vi "quiz3.4.vi"() -> ()   [LabVIEW 2017]
panel:
  out "Tab Control 2":enum32{"Login", "Menu", "Add", "delete"}(tab)
  in  "Ingresar 2":bool
  in  "Contraseña 2":string
  in  "Usuario 2":string
  in  "Delete Button 2":bool
  in  "Add Button 2":bool
  in  "Home Button 2":bool
  out "Cusuario 2":string
  in  "Previous Button 3":bool
  in  "AddContraseña 2":string
  in  "AddUsuario 2":string
  in  "Agregar 2":bool
  out "Agregado 2":bool
  in  "Cancel Button 2":bool
  in  "DeleteUsuario 3":string
  in  "Previous Button 4":bool
  out "text 2":string
  out "Tab Control":enum32{"Login", "Menu", "Add", "delete"}(tab)
  in  "Ingresar":bool
  in  "Contraseña":string
  in  "Usuario":string
  in  "Delete Button":bool
  in  "Add Button":bool
  in  "Home Button":bool
  out "Cusuario":string
  in  "Previous Button":bool
  in  "AddContraseña":string
  in  "AddUsuario":string
  in  "Agregar":bool
  out "Agregado":bool
  in  "Cancel Button":bool
  in  "DeleteUsuario":string
  in  "Previous Button 2":bool
  out "text":string
  # "USTED INGRESO CON EL USUARIO"
  # "USTED INGRESO CON EL USUARIO"
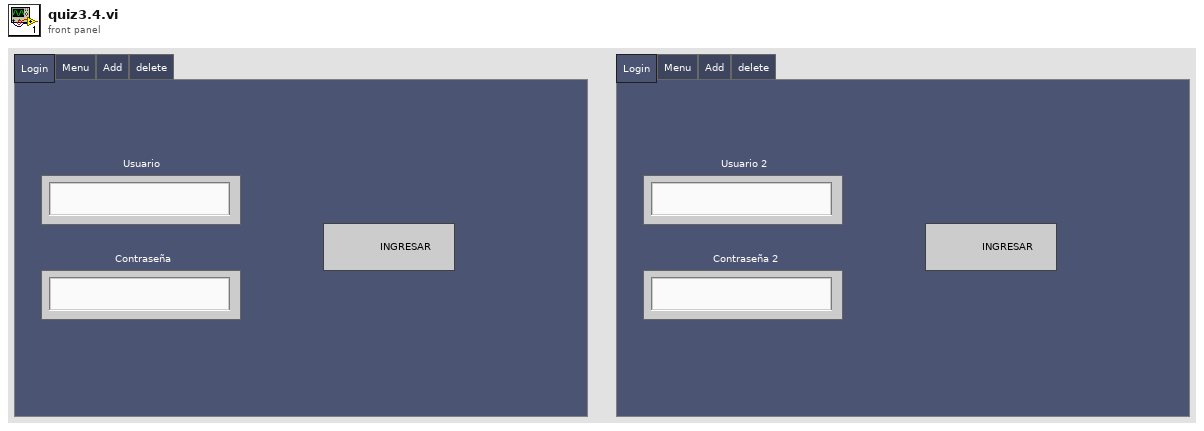
[diagram p1: front panel]
types:
  T1 = enum16{"open", "replace", "create", "open or create", "replace or create", "replace or create with confirmation"}
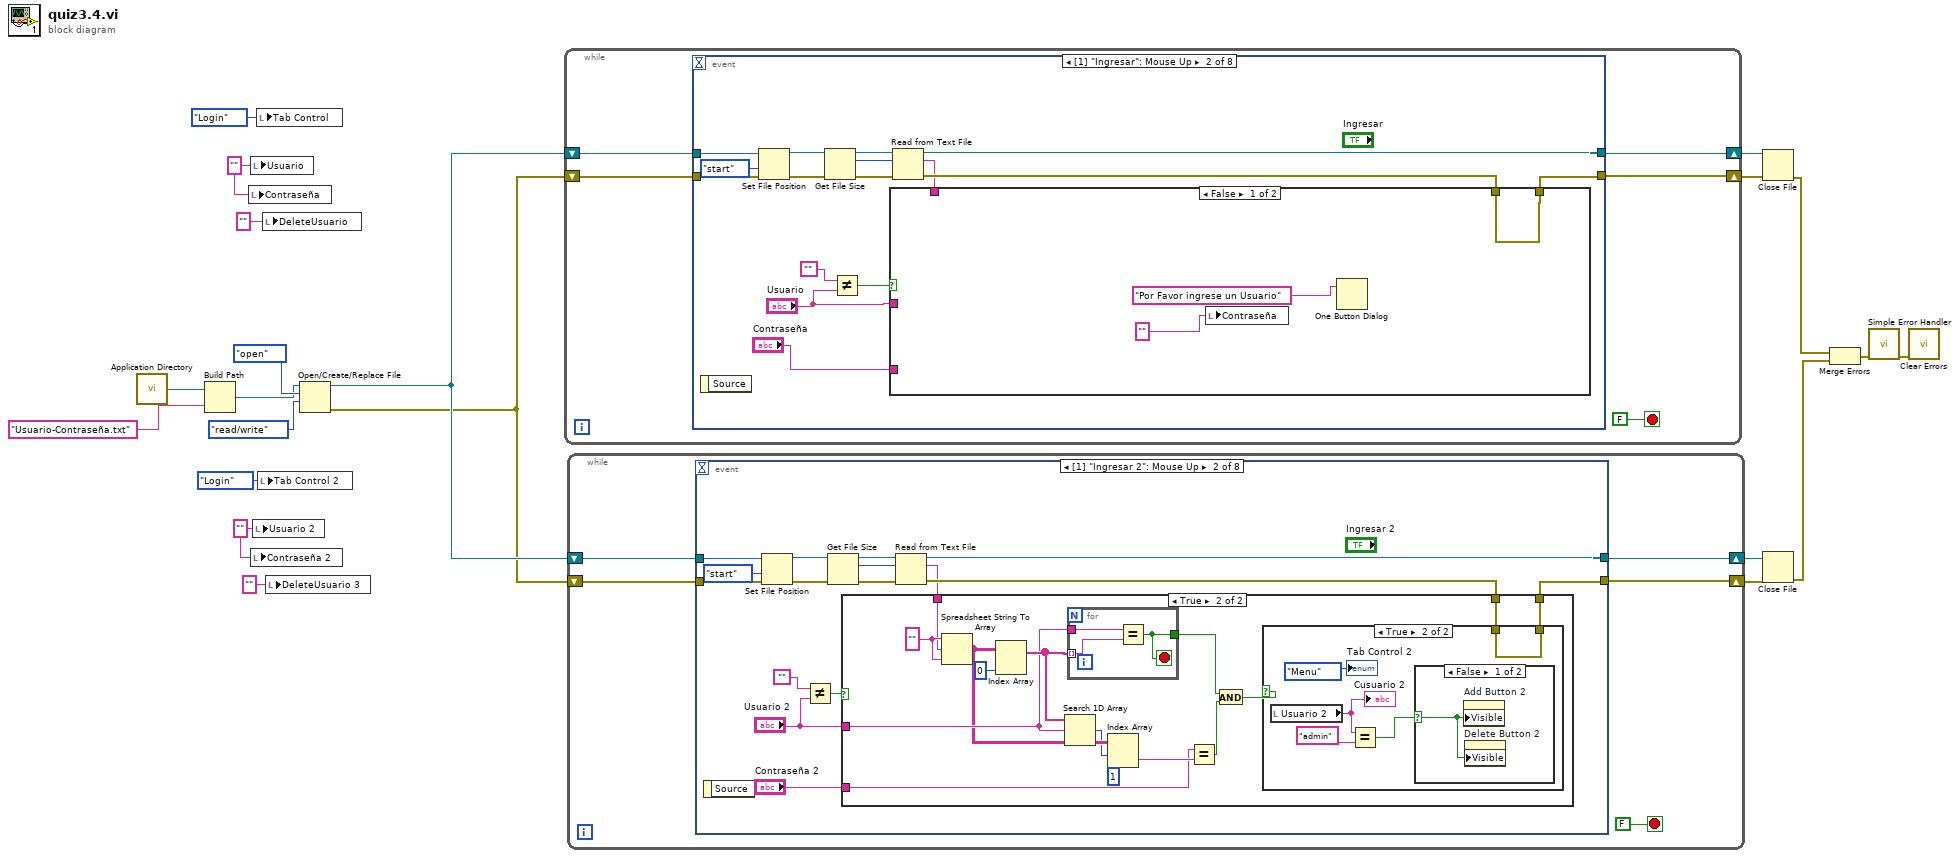
[diagram p0: block diagram]
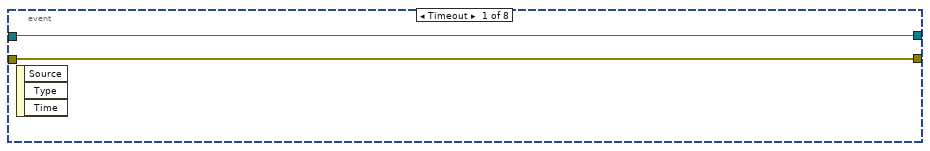
[diagram p2: hidden frame]
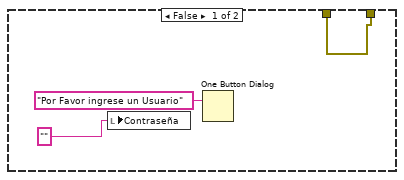
[diagram p3: hidden frame]
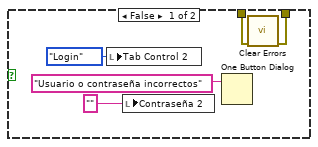
[diagram p4: hidden frame]
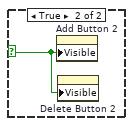
[diagram p5: hidden frame]
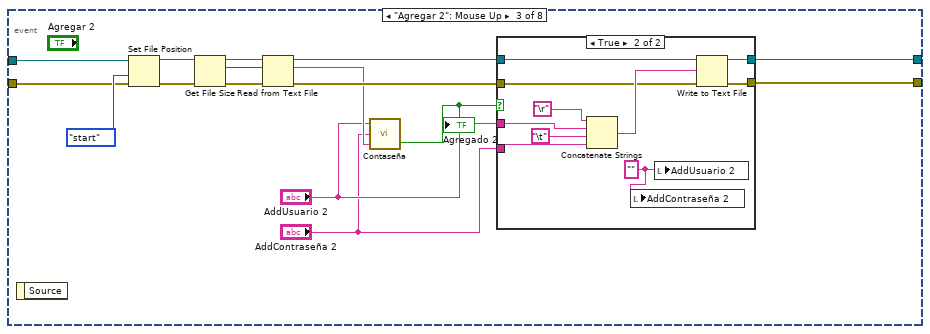
[diagram p6: hidden frame]
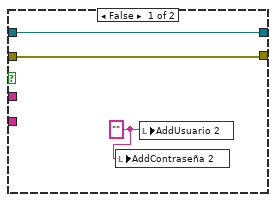
[diagram p7: hidden frame]
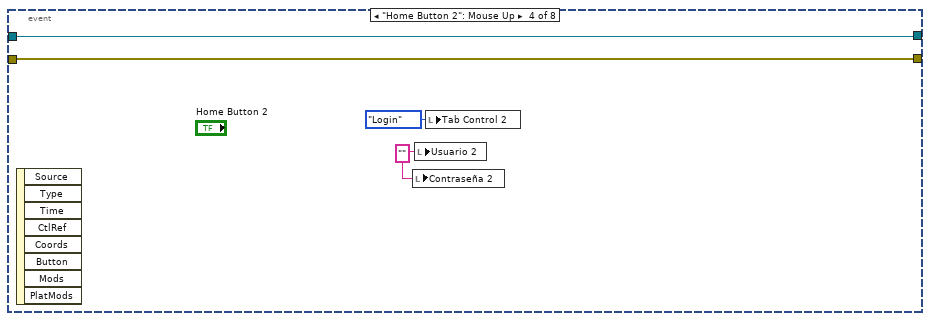
[diagram p8: hidden frame]
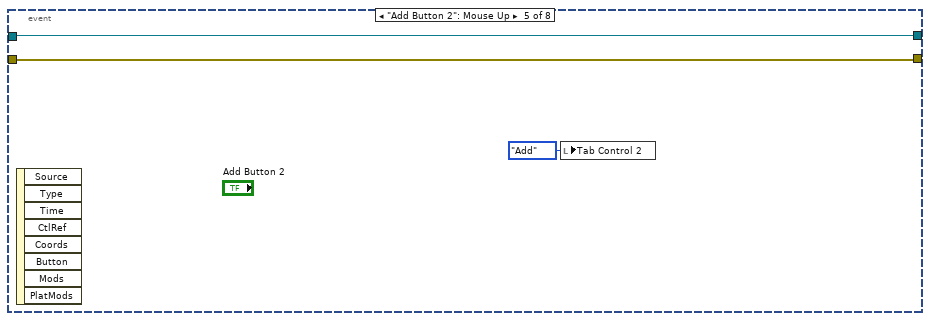
[diagram p9: hidden frame]
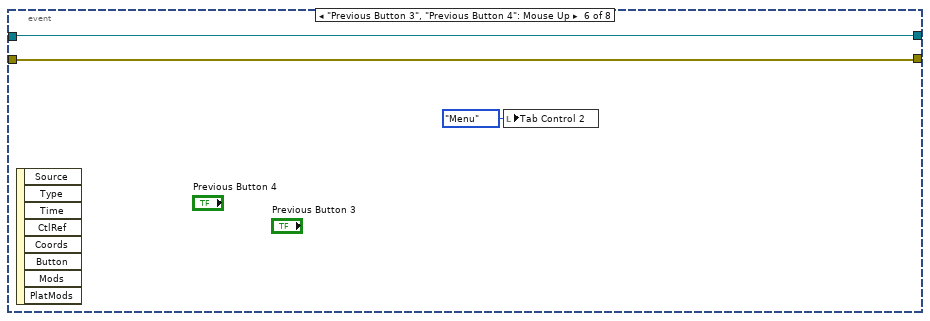
[diagram p10: hidden frame]
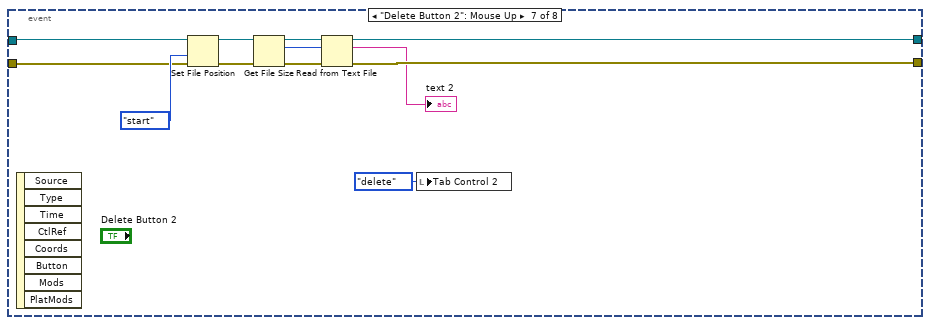
[diagram p11: hidden frame]
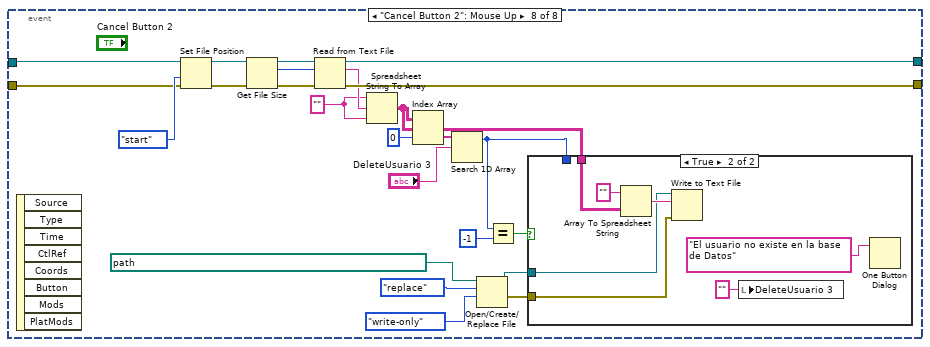
[diagram p12: hidden frame]
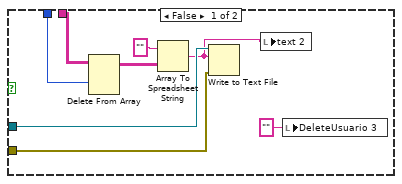
[diagram p13: hidden frame]
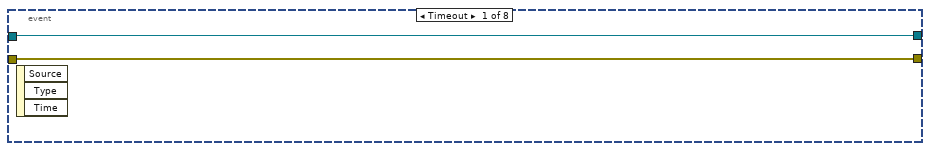
[diagram p14: hidden frame]
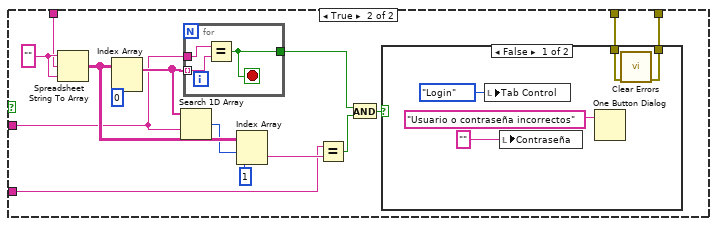
[diagram p15: hidden frame]
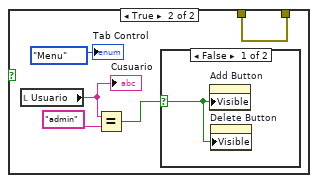
[diagram p16: hidden frame]
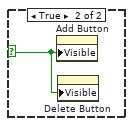
[diagram p17: hidden frame]
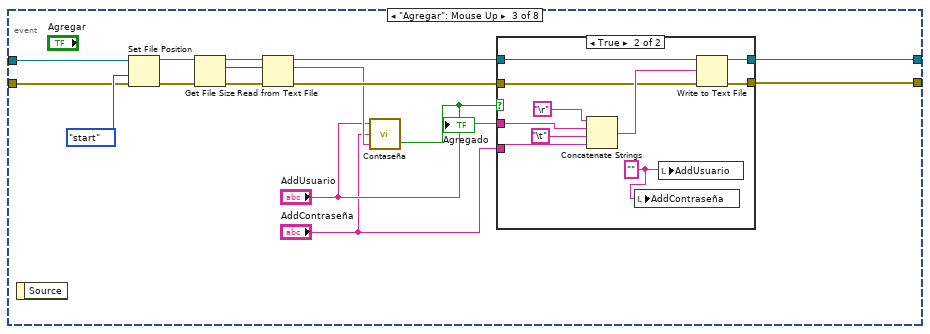
[diagram p18: hidden frame]
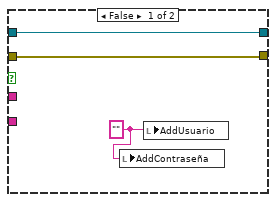
[diagram p19: hidden frame]
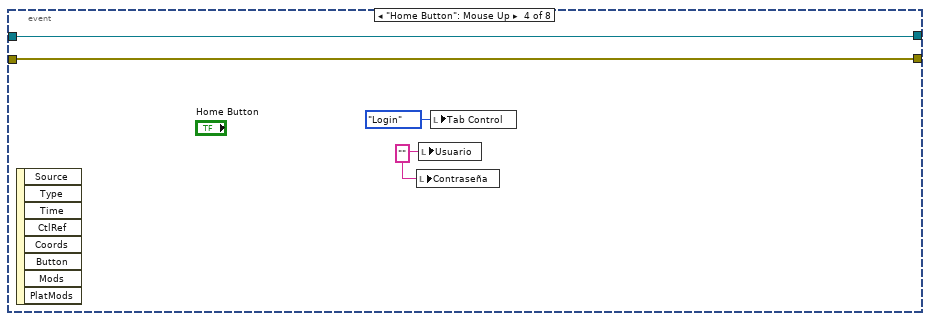
[diagram p20: hidden frame]
diagram:
  w1 = "" ("Usuario")
  w14 = "" ("Usuario")
  n1 = call <vilib>:"Application Directory.vi"() -> ("Application Directory"=w21:path)
  n2 = Build Path(base path=w21, name or relative path="Usuario-Contraseña.txt") -> (appended path=w15:path)
  n3 = local write "Contraseña"(w14) -> ()
  n4 = local write "Usuario"(w14) -> ()
  n5 = local write "Contraseña 2"(w1) -> ()
  n6 = local write "Usuario 2"(w1) -> ()
  n7 = local write "Tab Control"(enum32{"Login", "Menu", "Add", "delete"}."Login" ("Tab Control")) -> ()
  n8 = local write "Tab Control 2"(enum32{"Login", "Menu", "Add", "delete"}."Login" ("Tab Control")) -> ()
  n9 = local write "DeleteUsuario"("" ("DeleteUsuario 2")) -> ()
  n10 = local write "DeleteUsuario 3"("" ("DeleteUsuario 2")) -> ()
  n11 = Open/Create/Replace File(file path (use dialog)=w15, operation (0:open)=T1."open", access (0:read/write)=enum16{"read/write", "read-only", "write-only"}."read/write") -> (refnum out=w5:refnum<file>, error out=w4:errorcluster)  [unwired: 3 in, 1 out]
  n12 = while {
    shift-right: [w23] -> w11
    shift-left: w5 -> [w24]
    shift-right: [w22] -> w16
    shift-left: w4 -> [w25]
    stop <- FALSE stop-if-true
    n13 = event shown="[1] \"Ingresar\": Mouse Up" {
      selector: _ -> [_ _ _ _ _ _ _ _]
      dyn-events: _ -> [_ _ _ _ _ _ _ _]
      timeout: _ -> [_ _ _ _ _ _ _ _]
      tunnel: w25 -> [w27 w44 w81 w108 w112 w115 w119 w146]
      tunnel: [w28 w39 w93 w109 w113 w116 w120 w142] -> w23
      tunnel: [w27 w36 w92 w108 w112 w115 w118 w141] -> w22
      tunnel: w24 -> [w28 w38 w82 w109 w113 w116 w121 w145]
      event Timeout {
        n14 = event-data() -> ()  [unwired: 1 in, 3 out]
      }
      event "Ingresar": Mouse Up {
        n15 = event-data() -> ()  [unwired: 1 in, 1 out]
        n16 = Set File Position(refnum=w38, from (0:start)=enum16{"start", "end", "current"}."start", error in=w44) -> (refnum out=w42:refnum<file>, error out=w43:errorcluster)  [unwired: 1 in]
        n17 = Get File Size(file=w42, error in=w43) -> (refnum out=w34:refnum<file>, size (in bytes)=w41:i64, 0:w40:errorcluster)
        n18 = Not Equal?(x="", y="Usuario") -> (x != y?=w31:bool)
        n19 = Read from Text File(file (use dialog)=w34, count=w41, error in=w40) -> (refnum out=w39:refnum<file>, text=w33:string, error out=w37:errorcluster)  [unwired: 1 in, 1 out]
        n20 = case shown="False" w31 {
          tunnel: w37 -> [w47 w62]
          tunnel: [w47 w61] -> w36
          tunnel: w33 -> [_ w58]
          tunnel: "Usuario" -> [_ w49]
          tunnel: "Contraseña" -> [_ w48]
          frame False {
            n21 = local write "Contraseña"("" ("Usuario")) -> ()
            n22 = One Button Dialog(message="Por Favor ingrese un Usuario") -> ()  [unwired: 1 in, 1 out]
          }
          frame True {
            w59 = "" ("format string")
            n23 = Spreadsheet String To Array(format string=w59, spreadsheet string=w58, array type (2D Dbl)=w59) -> (array=w55:string[][])  [unwired: 1 in]
            n24 = Index Array(array=w55, index (col)=0 ("index")) -> (element=w56:string[])  [unwired: 1 in]
            n25 = Search 1D Array(1D array=w56, element=w49) -> (index of element=w52:i32)  [unwired: 1 in]
            n26 = for {
              tunnel: [w65] -> w57
              tunnel: w56 -> [w64] mode=indexing
              tunnel: w49 -> [w63]
              stop <- w65 stop-if-true
              n27 = Equal?(x=w63, y=w64) -> (x = y?=w65:bool)
            }
            n28 = Index Array(array=w55, index (row)=w52, index (col)=1 ("index")) -> (element=w50:string)
            n29 = Equal?(x=w48, y=w50) -> (x = y?=w54:bool)
            n30 = And(x=w57, y=w54) -> (x .and. y?=w60:bool)
            n31 = case shown="False" w60 {
              tunnel: [w68 w75] -> w61
              tunnel: w62 -> [w67 w75]
              frame False {
                n32 = local write "Tab Control"(enum32{"Login", "Menu", "Add", "delete"}."Login" ("Tab Control")) -> ()
                n33 = local write "Contraseña"("" ("Usuario")) -> ()
                n34 = One Button Dialog(message="Usuario o contraseña incorrectos") -> ()  [unwired: 1 in, 1 out]
                n35 = call <vilib>:"Clear Errors.vi"("error in (no error)"=w67) -> ("error out"=w68:errorcluster)  [unwired: 5 in, 1 out]
              }
              frame True {
                n36 = local read "Usuario"() -> (w73:string)
                "Cusuario" <- w73
                n37 = Equal?(x=w73, y="admin") -> (x = y?=w74:bool)
                n38 = case shown="False" w74 {
                  selector: w74 -> [w76 w77]
                  frame False {
                    n39 = property on="Add Button" class="Bool (strict)"("Visible"=w76) -> ()  [unwired: 2 in, 2 out]
                    n40 = property on="Delete Button" class="Bool (strict)"("Visible"=w76) -> ()  [unwired: 2 in, 2 out]
                  }
                  frame True {
                    n41 = property on="Add Button" class="Bool (strict)"("Visible"=w77) -> ()  [unwired: 2 in, 2 out]
                    n42 = property on="Delete Button" class="Bool (strict)"("Visible"=w77) -> ()  [unwired: 2 in, 2 out]
                  }
                }
                "Tab Control" <- enum32{"Login", "Menu", "Add", "delete"}."Menu" ("Tab Control")
              }
            }
          }
        }
      }
      event "Agregar": Mouse Up {
        n43 = event-data() -> ()  [unwired: 1 in, 1 out]
        n44 = Set File Position(refnum=w82, from (0:start)=enum16{"start", "end", "current"}."start", error in=w81) -> (refnum out=w89:refnum<file>, error out=w90:errorcluster)  [unwired: 1 in]
        n45 = Get File Size(file=w89, error in=w90) -> (refnum out=w86:refnum<file>, size (in bytes)=w88:i64, 0:w87:errorcluster)
        n46 = Read from Text File(file (use dialog)=w86, count=w88, error in=w87) -> (refnum out=w84:refnum<file>, text=w80:string, error out=w83:errorcluster)  [unwired: 1 in, 1 out]
        n47 = call "Contaseña.vi"("spreadsheet string"=w80, "AddContraseña"="AddContraseña", "addUsuario"="AddUsuario") -> ("result"=w91:bool)  [unwired: 1 out]
        "Agregado" <- w91
        n48 = case shown="True" w91 {
          tunnel: [w96 w106] -> w93
          tunnel: [w95 w105] -> w92
          tunnel: w84 -> [w96 w101]
          tunnel: w83 -> [w95 w100]
          tunnel: "AddUsuario" -> [_ w99]
          tunnel: "AddContraseña" -> [_ w98]
          frame False {
            w94 = "" ("Usuario")
            n49 = local write "AddContraseña"(w94) -> ()
            n50 = local write "AddUsuario"(w94) -> ()
          }
          frame True {
            w97 = "" ("Usuario")
            n51 = Concatenate Strings("\r", w99, "\t", w98) -> (w104:string)
            n52 = local write "AddContraseña"(w97) -> ()
            n53 = local write "AddUsuario"(w97) -> ()
            n54 = Write to Text File(file (use dialog)=w101, text=w104, error in=w100) -> (refnum out=w106:refnum<file>, error out=w105:errorcluster)  [unwired: 1 in, 1 out]
          }
        }
      }
      event "Home Button": Mouse Up {
        w110 = "" ("Usuario")
        n55 = event-data() -> ()  [unwired: 1 in, 8 out]
        n56 = local write "Contraseña"(w110) -> ()
        n57 = local write "Usuario"(w110) -> ()
        n58 = local write "Tab Control"(enum32{"Login", "Menu", "Add", "delete"}."Login" ("Tab Control")) -> ()
      }
      event "Add Button": Mouse Up {
        n59 = event-data() -> ()  [unwired: 1 in, 8 out]
        n60 = local write "Tab Control"(enum32{"Login", "Menu", "Add", "delete"}."Add" ("Tab Control")) -> ()
      }
      event "Previous Button", "Previous Button 2": Mouse Up {
        n61 = event-data() -> ()  [unwired: 1 in, 8 out]
        n62 = local write "Tab Control"(enum32{"Login", "Menu", "Add", "delete"}."Menu" ("Tab Control")) -> ()
      }
      event "Delete Button": Mouse Up {
        n63 = event-data() -> ()  [unwired: 1 in, 8 out]
        n64 = Set File Position(refnum=w121, from (0:start)=enum16{"start", "end", "current"}."start", error in=w119) -> (refnum out=w126:refnum<file>, error out=w127:errorcluster)  [unwired: 1 in]
        n65 = Get File Size(file=w126, error in=w127) -> (refnum out=w123:refnum<file>, size (in bytes)=w125:i64, 0:w124:errorcluster)
        n66 = Read from Text File(file (use dialog)=w123, count=w125, error in=w124) -> (refnum out=w120:refnum<file>, text=→"text":string, error out=w118:errorcluster)  [unwired: 1 in, 1 out]
        n67 = local write "Tab Control"(enum32{"Login", "Menu", "Add", "delete"}."delete" ("Tab Control")) -> ()
      }
      event "Cancel Button": Mouse Up {
        w138 = "" ("format string")
        n68 = event-data() -> ()  [unwired: 1 in, 8 out]
        n69 = Set File Position(refnum=w145, from (0:start)=enum16{"start", "end", "current"}."start", error in=w146) -> (refnum out=w151:refnum<file>, error out=w152:errorcluster)  [unwired: 1 in]
        n70 = Get File Size(file=w151, error in=w152) -> (refnum out=w148:refnum<file>, size (in bytes)=w150:i64, 0:w149:errorcluster)
        n71 = Read from Text File(file (use dialog)=w148, count=w150, error in=w149) -> (refnum out=w142:refnum<file>, text=w139:string, error out=w141:errorcluster)  [unwired: 1 in, 1 out]
        n72 = Spreadsheet String To Array(format string=w138, spreadsheet string=w139, array type (2D Dbl)=w138) -> (array=w134:string[][])  [unwired: 1 in]
        n73 = Index Array(array=w134, index (col)=0 ("disabled index (col)")) -> (element=w136:string[])  [unwired: 1 in]
        n74 = Search 1D Array(1D array=w136, element="DeleteUsuario") -> (index of element=w130:i32)  [unwired: 1 in]
        n75 = Open/Create/Replace File(file path (use dialog)=path "D:/2019-1/Programacion 2/quiz 3/Usuario-Contraseña.txt", operation (0:open)=T1."replace", access (0:read/write)=enum16{"read/write", "read-only", "write-only"}."write-only") -> (refnum out=w133:refnum<file>, error out=w132:errorcluster)  [unwired: 3 in, 1 out]
        n76 = Equal?(x=w130, y=-1) -> (x = y?=w131:bool)
        n77 = case shown="True" w131 {
          tunnel: w134 -> [w160 w163]
          tunnel: w130 -> [w159 _]
          tunnel: w133 -> [w157 w162]
          tunnel: w132 -> [w156 w161]
          frame False {
            n78 = Delete From Array(array=w160, index (row)=w159) -> (array with subset deleted=w158:string[][])  [unwired: 2 in, 1 out]
            n79 = Array To Spreadsheet String(array=w158, 3:"" ("format string")) -> (spreadsheet string=w154:string)  [unwired: 1 in]
            n80 = Write to Text File(file (use dialog)=w157, text=w154, error in=w156) -> ()  [unwired: 1 in, 3 out]
            n81 = local write "text"(w154) -> ()
            n82 = local write "DeleteUsuario"("" ("DeleteUsuario 2")) -> ()
          }
          frame True {
            n83 = Array To Spreadsheet String(array=w163, 3:"" ("format string")) -> (spreadsheet string=w165:string)  [unwired: 1 in]
            n84 = Write to Text File(file (use dialog)=w162, text=w165, error in=w161) -> ()  [unwired: 1 in, 3 out]
            n85 = local write "DeleteUsuario"("" ("DeleteUsuario 2")) -> ()
            n86 = One Button Dialog(message="El usuario no existe en la base de Datos") -> ()  [unwired: 1 in, 1 out]
          }
        }
      }
    }
  }
  n87 = while {
    shift-right: [w169] -> w6
    shift-left: w5 -> [w170]
    shift-right: [w168] -> w7
    shift-left: w4 -> [w171]
    stop <- FALSE stop-if-true
    n88 = event shown="[1] \"Ingresar 2\": Mouse Up" {
      selector: _ -> [_ _ _ _ _ _ _ _]
      dyn-events: _ -> [_ _ _ _ _ _ _ _]
      timeout: _ -> [_ _ _ _ _ _ _ _]
      tunnel: w171 -> [w173 w190 w227 w254 w258 w261 w265 w292]
      tunnel: [w174 w185 w239 w255 w259 w262 w266 w288] -> w169
      tunnel: [w173 w182 w238 w254 w258 w261 w264 w287] -> w168
      tunnel: w170 -> [w174 w184 w228 w255 w259 w262 w267 w291]
      event Timeout {
        n89 = event-data() -> ()  [unwired: 1 in, 3 out]
      }
      event "Ingresar 2": Mouse Up {
        n90 = event-data() -> ()  [unwired: 1 in, 1 out]
        n91 = Set File Position(refnum=w184, from (0:start)=enum16{"start", "end", "current"}."start", error in=w190) -> (refnum out=w188:refnum<file>, error out=w189:errorcluster)  [unwired: 1 in]
        n92 = Not Equal?(x="", y="Usuario 2") -> (x != y?=w176:bool)
        n93 = Get File Size(file=w188, error in=w189) -> (refnum out=w180:refnum<file>, size (in bytes)=w187:i64, 0:w186:errorcluster)
        n94 = Read from Text File(file (use dialog)=w180, count=w187, error in=w186) -> (refnum out=w185:refnum<file>, text=w179:string, error out=w183:errorcluster)  [unwired: 1 in, 1 out]
        n95 = case shown="True" w176 {
          tunnel: w183 -> [w193 w208]
          tunnel: [w193 w207] -> w182
          tunnel: w179 -> [_ w204]
          tunnel: "Usuario 2" -> [_ w201]
          tunnel: "Contraseña 2" -> [_ w194]
          frame False {
            n96 = local write "Contraseña"("" ("Usuario")) -> ()
            n97 = One Button Dialog(message="Por Favor ingrese un Usuario") -> ()  [unwired: 1 in, 1 out]
          }
          frame True {
            w205 = "" ("format string")
            n98 = Spreadsheet String To Array(format string=w205, spreadsheet string=w204, array type (2D Dbl)=w205) -> (array=w200:string[][])  [unwired: 1 in]
            n99 = Index Array(array=w200, index (col)=0 ("index")) -> (element=w202:string[])  [unwired: 1 in]
            n100 = Search 1D Array(1D array=w202, element=w201) -> (index of element=w197:i32)  [unwired: 1 in]
            n101 = for {
              tunnel: w201 -> [w211]
              tunnel: [w210] -> w203
              tunnel: w202 -> [w209] mode=indexing
              stop <- w210 stop-if-true
              n102 = Equal?(x=w211, y=w209) -> (x = y?=w210:bool)
            }
            n103 = Index Array(array=w200, index (row)=w197, index (col)=1 ("index")) -> (element=w195:string)
            n104 = Equal?(x=w194, y=w195) -> (x = y?=w199:bool)
            n105 = And(x=w203, y=w199) -> (x .and. y?=w206:bool)
            n106 = case shown="True" w206 {
              tunnel: [w214 w221] -> w207
              tunnel: w208 -> [w213 w221]
              frame False {
                n107 = local write "Tab Control 2"(enum32{"Login", "Menu", "Add", "delete"}."Login" ("Tab Control")) -> ()
                n108 = local write "Contraseña 2"("" ("Usuario")) -> ()
                n109 = One Button Dialog(message="Usuario o contraseña incorrectos") -> ()  [unwired: 1 in, 1 out]
                n110 = call <vilib>:"Clear Errors.vi"("error in (no error)"=w213) -> ("error out"=w214:errorcluster)  [unwired: 5 in, 1 out]
              }
              frame True {
                n111 = local read "Usuario 2"() -> (w219:string)
                "Cusuario 2" <- w219
                n112 = Equal?(x=w219, y="admin") -> (x = y?=w220:bool)
                n113 = case shown="False" w220 {
                  selector: w220 -> [w222 w223]
                  frame False {
                    n114 = property on="Add Button 2" class="Bool (strict)"("Visible"=w222) -> ()  [unwired: 2 in, 2 out]
                    n115 = property on="Delete Button 2" class="Bool (strict)"("Visible"=w222) -> ()  [unwired: 2 in, 2 out]
                  }
                  frame True {
                    n116 = property on="Add Button 2" class="Bool (strict)"("Visible"=w223) -> ()  [unwired: 2 in, 2 out]
                    n117 = property on="Delete Button 2" class="Bool (strict)"("Visible"=w223) -> ()  [unwired: 2 in, 2 out]
                  }
                }
                "Tab Control 2" <- enum32{"Login", "Menu", "Add", "delete"}."Menu" ("Tab Control")
              }
            }
          }
        }
      }
      event "Agregar 2": Mouse Up {
        n118 = event-data() -> ()  [unwired: 1 in, 1 out]
        n119 = Set File Position(refnum=w228, from (0:start)=enum16{"start", "end", "current"}."start", error in=w227) -> (refnum out=w235:refnum<file>, error out=w236:errorcluster)  [unwired: 1 in]
        n120 = Get File Size(file=w235, error in=w236) -> (refnum out=w232:refnum<file>, size (in bytes)=w234:i64, 0:w233:errorcluster)
        n121 = Read from Text File(file (use dialog)=w232, count=w234, error in=w233) -> (refnum out=w230:refnum<file>, text=w226:string, error out=w229:errorcluster)  [unwired: 1 in, 1 out]
        n122 = call "Contaseña.vi"("spreadsheet string"=w226, "AddContraseña"="AddContraseña 2", "addUsuario"="AddUsuario 2") -> ("result"=w237:bool)  [unwired: 1 out]
        "Agregado 2" <- w237
        n123 = case shown="True" w237 {
          tunnel: [w242 w252] -> w239
          tunnel: [w241 w251] -> w238
          tunnel: w230 -> [w242 w247]
          tunnel: w229 -> [w241 w246]
          tunnel: "AddUsuario 2" -> [_ w245]
          tunnel: "AddContraseña 2" -> [_ w244]
          frame False {
            w240 = "" ("Usuario")
            n124 = local write "AddContraseña 2"(w240) -> ()
            n125 = local write "AddUsuario 2"(w240) -> ()
          }
          frame True {
            w243 = "" ("Usuario")
            n126 = Concatenate Strings("\r", w245, "\t", w244) -> (w250:string)
            n127 = local write "AddContraseña 2"(w243) -> ()
            n128 = local write "AddUsuario 2"(w243) -> ()
            n129 = Write to Text File(file (use dialog)=w247, text=w250, error in=w246) -> (refnum out=w252:refnum<file>, error out=w251:errorcluster)  [unwired: 1 in, 1 out]
          }
        }
      }
      event "Home Button 2": Mouse Up {
        w256 = "" ("Usuario")
        n130 = event-data() -> ()  [unwired: 1 in, 8 out]
        n131 = local write "Contraseña 2"(w256) -> ()
        n132 = local write "Usuario 2"(w256) -> ()
        n133 = local write "Tab Control 2"(enum32{"Login", "Menu", "Add", "delete"}."Login" ("Tab Control")) -> ()
      }
      event "Add Button 2": Mouse Up {
        n134 = event-data() -> ()  [unwired: 1 in, 8 out]
        n135 = local write "Tab Control 2"(enum32{"Login", "Menu", "Add", "delete"}."Add" ("Tab Control")) -> ()
      }
      event "Previous Button 3", "Previous Button 4": Mouse Up {
        n136 = event-data() -> ()  [unwired: 1 in, 8 out]
        n137 = local write "Tab Control 2"(enum32{"Login", "Menu", "Add", "delete"}."Menu" ("Tab Control")) -> ()
      }
      event "Delete Button 2": Mouse Up {
        n138 = event-data() -> ()  [unwired: 1 in, 8 out]
        n139 = Set File Position(refnum=w267, from (0:start)=enum16{"start", "end", "current"}."start", error in=w265) -> (refnum out=w272:refnum<file>, error out=w273:errorcluster)  [unwired: 1 in]
        n140 = Get File Size(file=w272, error in=w273) -> (refnum out=w269:refnum<file>, size (in bytes)=w271:i64, 0:w270:errorcluster)
        n141 = Read from Text File(file (use dialog)=w269, count=w271, error in=w270) -> (refnum out=w266:refnum<file>, text=→"text 2":string, error out=w264:errorcluster)  [unwired: 1 in, 1 out]
        n142 = local write "Tab Control 2"(enum32{"Login", "Menu", "Add", "delete"}."delete" ("Tab Control")) -> ()
      }
      event "Cancel Button 2": Mouse Up {
        w284 = "" ("format string")
        n143 = event-data() -> ()  [unwired: 1 in, 8 out]
        n144 = Set File Position(refnum=w291, from (0:start)=enum16{"start", "end", "current"}."start", error in=w292) -> (refnum out=w297:refnum<file>, error out=w298:errorcluster)  [unwired: 1 in]
        n145 = Get File Size(file=w297, error in=w298) -> (refnum out=w294:refnum<file>, size (in bytes)=w296:i64, 0:w295:errorcluster)
        n146 = Read from Text File(file (use dialog)=w294, count=w296, error in=w295) -> (refnum out=w288:refnum<file>, text=w285:string, error out=w287:errorcluster)  [unwired: 1 in, 1 out]
        n147 = Spreadsheet String To Array(format string=w284, spreadsheet string=w285, array type (2D Dbl)=w284) -> (array=w280:string[][])  [unwired: 1 in]
        n148 = Index Array(array=w280, index (col)=0 ("disabled index (col)")) -> (element=w282:string[])  [unwired: 1 in]
        n149 = Search 1D Array(1D array=w282, element="DeleteUsuario 3") -> (index of element=w276:i32)  [unwired: 1 in]
        n150 = Open/Create/Replace File(file path (use dialog)=path "D:/2019-1/Programacion 2/quiz 3/Usuario-Contraseña.txt", operation (0:open)=T1."replace", access (0:read/write)=enum16{"read/write", "read-only", "write-only"}."write-only") -> (refnum out=w279:refnum<file>, error out=w278:errorcluster)  [unwired: 3 in, 1 out]
        n151 = Equal?(x=w276, y=-1) -> (x = y?=w277:bool)
        n152 = case shown="True" w277 {
          tunnel: w280 -> [w306 w309]
          tunnel: w276 -> [w305 _]
          tunnel: w279 -> [w303 w308]
          tunnel: w278 -> [w302 w307]
          frame False {
            n153 = Delete From Array(array=w306, index (row)=w305) -> (array with subset deleted=w304:string[][])  [unwired: 2 in, 1 out]
            n154 = Array To Spreadsheet String(array=w304, 3:"" ("format string")) -> (spreadsheet string=w300:string)  [unwired: 1 in]
            n155 = Write to Text File(file (use dialog)=w303, text=w300, error in=w302) -> ()  [unwired: 1 in, 3 out]
            n156 = local write "text 2"(w300) -> ()
            n157 = local write "DeleteUsuario 3"("" ("DeleteUsuario 2")) -> ()
          }
          frame True {
            n158 = Array To Spreadsheet String(array=w309, 3:"" ("format string")) -> (spreadsheet string=w311:string)  [unwired: 1 in]
            n159 = Write to Text File(file (use dialog)=w308, text=w311, error in=w307) -> ()  [unwired: 1 in, 3 out]
            n160 = local write "DeleteUsuario 3"("" ("DeleteUsuario 2")) -> ()
            n161 = One Button Dialog(message="El usuario no existe en la base de Datos") -> ()  [unwired: 1 in, 1 out]
          }
        }
      }
    }
  }
  n162 = Close File(refnum=w11, error in=w16) -> (error out=w9:errorcluster)  [unwired: 1 out]
  n163 = Close File(refnum=w6, error in=w7) -> (error out=w8:errorcluster)  [unwired: 1 out]
  n164 = Merge Errors(w9, w8) -> (w10:errorcluster)
  n165 = call <vilib>:"Simple Error Handler.vi"("error in (no error)"=w10) -> ("error out"=w17:errorcluster)  [unwired: 4 in, 4 out]
  n166 = call <vilib>:"Clear Errors.vi"("error in (no error)"=w17) -> ()  [unwired: 5 in, 2 out]
